vi "Convert Assert Event Data to Test Case - Error - Message.vi"() -> ()   [LabVIEW 2013, in "JUnit Conversion Tests.lvlib"]
uses:
  JUnit Conversion Tests.lvlib
  <vilib>/addons/_JKI Toolkits/Caraya/classes/Test Result/Assert Event Data (Extended).ctl
  JUnit XML/Test Case/Test Case.lvclass/Test Case.ctl
  JUnit XML/Test Case/Read Message.vi
  <vilib>/addons/_JKI Toolkits/Caraya/classes/Assert/Assert Equal Value_Variant.vi
  JUnit Conversion/JUnit Conversion.lvlib
  <vilib>/addons/_JKI Toolkits/Caraya/classes/Test Result/Test Result.lvclass
  <vilib>/addons/_JKI Toolkits/Caraya/classes/Assert/Assert.lvclass
  <vilib>/addons/_JKI Toolkits/Caraya/classes/Test/Test.lvclass
  JUnit XML/Test Case/Test Case.lvclass
panel:
  out "error out":errorcluster
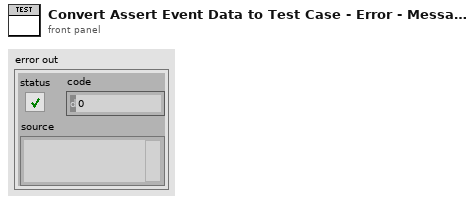
[diagram p1: front panel]
types:
  T1 = typedef "Caraya.lvlib/Test Result.lvclass/Assert Event Data (Extended).ctl" = cluster{"name":string, "passed":bool, "call-chain":string[], "test-error":errorcluster, "timestamp":timestamp, "assert-id":string, "test-id":string, "time":dbl, "message":string, "properties":variant, "measurements":variant, "user-defined":variant}
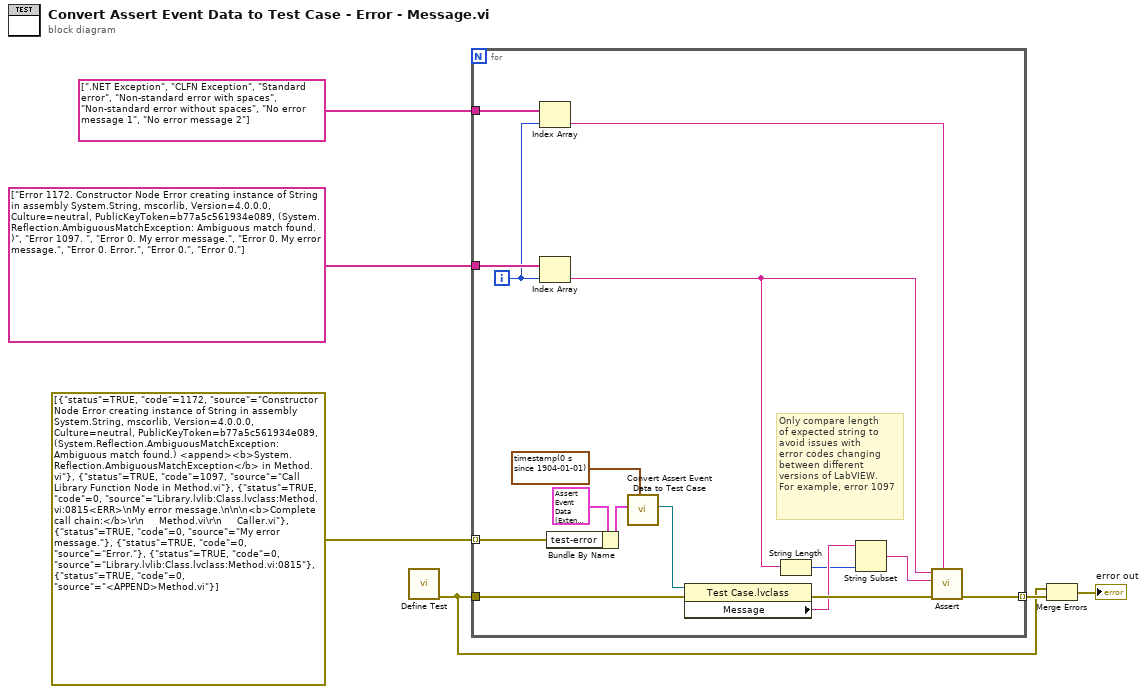
[diagram p0: block diagram]
diagram:
  n1 = call <vilib>:"Define Test.vi"() -> ("error out"=w4:errorcluster)  [unwired: 10 in, 1 out]
  n2 = for {
    tunnel: [w22] -> w6 mode=indexing
    tunnel: w4 -> [w21]
    tunnel: string[] ["Error 1172. Constructor Node Error creating instance of String in assembly System.String, mscorlib, Version=4.0.0.0, Culture=neutral, PublicKeyToken=b77a5c561934e089, (System.Reflection.AmbiguousMatchException: Ambiguous match found.)", "Error 1097. ", "Error 0. My error message.", "Error 0. My error message.", "Error 0. Error.", "Error 0.", "Error 0."] -> [w15]
    tunnel: errorcluster[] [{"status"=TRUE, "code"=1172, "source"="Constructor Node Error creating instance of String in assembly System.String, mscorlib, Version=4.0.0.0, Culture=neutral, PublicKeyToken=b77a5c561934e089, (System.Reflection.AmbiguousMatchException: Ambiguous match found.) <append><b>System.Reflection.AmbiguousMatchException</b> in Method.vi"}, {"status"=TRUE, "code"=1097, "source"="Call Library Function Node in Method.vi"}, {"status"=TRUE, "code"=0, "source"="Library.lvlib:Class.lvclass:Method.vi:0815<ERR>\nMy error message.\n\n\n<b>Complete call chain:</b>\r\n     Method.vi\r\n     Caller.vi"}, {"status"=TRUE, "code"=0, "source"="My error message."}, {"status"=TRUE, "code"=0, "source"="Error."}, {"status"=TRUE, "code"=0, "source"="Library.lvlib:Class.lvclass:Method.vi:0815"}, {"status"=TRUE, "code"=0, "source"="<APPEND>Method.vi"}] -> [w14] mode=indexing
    tunnel: string[] [".NET Exception", "CLFN Exception", "Standard error", "Non-standard error with spaces", "Non-standard error without spaces", "No error message 1", "No error message 2"] -> [w13]
    i -> [w11]
    # "Only compare length\nof expected string to\navoid issues with\nerror codes changing\nbetween different\nversions of LabVIEW.\nFor example, error 1097"
    n3 = Index Array(array=w13, index=w11) -> (element=w12:string)
    n4 = Index Array(array=w15, index=w11) -> (element=w7:string)
    n5 = Bundle By Name(cluster=T1 {"name"="", "passed"=FALSE, "call-chain"=[], "test-error"={"status"=FALSE, "code"=0, "source"=""}, "timestamp"=timestamp(0 s since 1904-01-01), "assert-id"="", "test-id"="", "time"=-1.0, "message"="", "properties"=variant, "measurements"=variant, "user-defined"=variant} ("Assert Event Data"), "test-error"=w14) -> (w19:T1)
    n6 = call "Convert Assert Event Data to Test Case.vi"("Start Time"=timestamp(0 s since 1904-01-01), "Assert Event Data"=w19) -> ("Test Case"=w18:refnum<class "Test Case.lvclass">)  [unwired: 9 in]
    n7 = property on="Property Node" class="Test Case.lvclass"(reference=w18, error in=w21) -> (error out=w17:errorcluster, "Message"=w10:string)  [unwired: 1 out]
    n8 = String Length(string=w7) -> (length=w8:i32)
    n9 = String Subset(string=w10, length (rest)=w8) -> (substring=w9:string)  [unwired: 1 in]
    n10 = call-poly <vilib>:"Assert.vi"("Label"=w12, "error in (no error)"=w17, "Y"=w9, "X"=w7) -> ("error out"=w22:errorcluster)  [unwired: 6 in, 1 out]
  }
  n11 = Merge Errors(w4, w6) -> (→"error out":errorcluster)
